vi "Test Serialize Clusters.vi"(8 "error in (no error)":errorcluster) -> (0 "error out":errorcluster)   [LabVIEW 2013]
uses:
  src/Serializer/JSON Serializer/JSON Serializer.lvclass
  <vilib>/addons/_JKI Toolkits/Caraya/classes/Test/Test.lvclass
  <vilib>/addons/_JKI Toolkits/Caraya/classes/Assert/Assert.lvclass
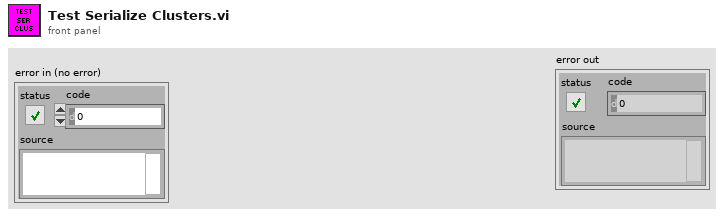
[diagram p1: front panel]
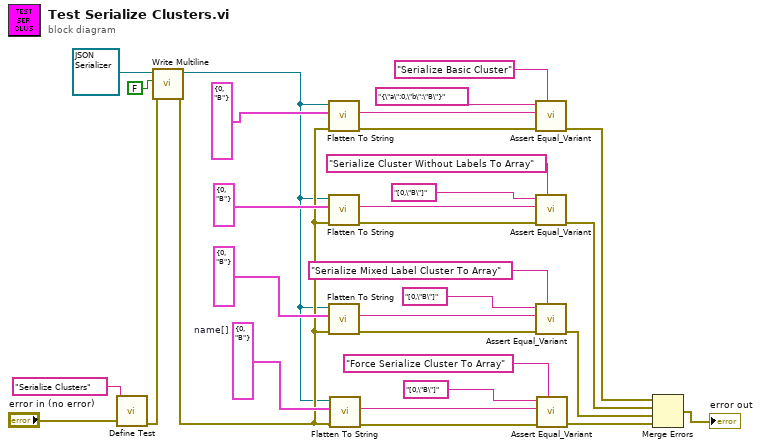
[diagram p0: block diagram]
diagram:
  w6 = cluster{"a":i32, "b":string} {"a"=0, "b"="B"}  # name[]
  n1 = call <vilib>:"Define Test.vi"("error in (no error)"="error in (no error)", "Label (VI Title)"="Serialize Clusters") -> ("error out"=w17:errorcluster)  [unwired: 9 in]
  n2 = call-dynamic "Write Multiline.vi"("error in (no error)"=w17, "Multiline"=FALSE, "JSON Serializer in"=refnum<class "JSON Serializer.lvclass"> refnum ("JKI JSON Serialization.lvlib:JSON Serializer.lvclass")) -> ("error out"=w3:errorcluster, "JSON Serializer out"=w2:refnum<class "JSON Serializer.lvclass">)  [unwired: 7 in]
  n3 = call-dynamic "Flatten To String.vi"("error in (no error)"=w3, "Variant"=cluster{"a":i32, "b":string} {"a"=0, "b"="B"}, "JSON Serializer in"=w2) -> ("error out"=w27:errorcluster, "String"=w26:string)  [unwired: 6 in, 1 out]
  n4 = call-dynamic "Flatten To String.vi"("error in (no error)"=w3, "Variant"=cluster{i32, string} {0, "B"}, "JSON Serializer in"=w2) -> ("error out"=w30:errorcluster, "String"=w29:string)  [unwired: 6 in, 1 out]
  n5 = call-dynamic "Flatten To String.vi"("error in (no error)"=w3, "Variant"=cluster{"a":i32, string} {"a"=0, "B"}, "JSON Serializer in"=w2) -> ("error out"=w15:errorcluster, "String"=w10:string)  [unwired: 6 in, 1 out]
  n6 = call-dynamic "Flatten To String.vi"("error in (no error)"=w3, "Variant"=w6, "JSON Serializer in"=w2) -> ("error out"=w7:errorcluster, "String"=w5:string)  [unwired: 6 in, 1 out]
  n7 = call <vilib>:"Assert Equal_Variant.vi"("Label"="Serialize Basic Cluster", "error in (no error)"=w27, "Y"=w26, "X"="{\"a\":0,\"b\":\"B\"}") -> ("error out"=w20:errorcluster)  [unwired: 7 in]
  n8 = call <vilib>:"Assert Equal_Variant.vi"("Label"="Serialize Cluster Without Labels To Array", "error in (no error)"=w30, "Y"=w29, "X"="[0,\"B\"]") -> ("error out"=w21:errorcluster)  [unwired: 7 in]
  n9 = call <vilib>:"Assert Equal_Variant.vi"("Label"="Serialize Mixed Label Cluster To Array", "error in (no error)"=w15, "Y"=w10, "X"="[0,\"B\"]") -> ("error out"=w22:errorcluster)  [unwired: 7 in]
  n10 = call <vilib>:"Assert Equal_Variant.vi"("Label"="Force Serialize Cluster To Array", "error in (no error)"=w7, "Y"=w5, "X"="[0,\"B\"]") -> ("error out"=w1:errorcluster)  [unwired: 7 in]
  n11 = Merge Errors(w20, w21, w22, w1) -> (→"error out":errorcluster)
